vi "GlobalDisplayIndex.vi"() -> ()   [LabVIEW 2013]
panel:
  in  "display speed":string[](array[combo])
  out "display canID":dbl[](array[numeric])
  out "display address":dbl[](array[numeric])
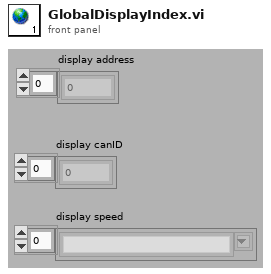
[diagram p1: front panel]
diagram:
